vi "IQxstream_Init.vi"(4 "WaveformBW":u16(ring)=1 items=["20 MHz", "100 MHz"], 6 "Transmission":u16(ring) items=["CW", "Waveform"], 8 "error in (no error)":errorcluster, 9 "TRXmode":u16(ring) items=["Tx", "Rx"], 10 "Freq":dbl=3.5 format="%#_13g", 11 "VISA resource name":refnum<visa-resource-name>="LitePoint_IQxstream") -> (0 "error out":errorcluster, 2 "read buffer":string="LitePoint,IQxstream-5G,IQ132CA8300,1.11.2\n", 3 "VISA resource name out":refnum<visa-resource-name>="LitePoint_IQxstream")   [LabVIEW 2020, in "LitePoints.lvlib"]
uses:
  LitePoints.lvlib
panel:
  # "GHz"
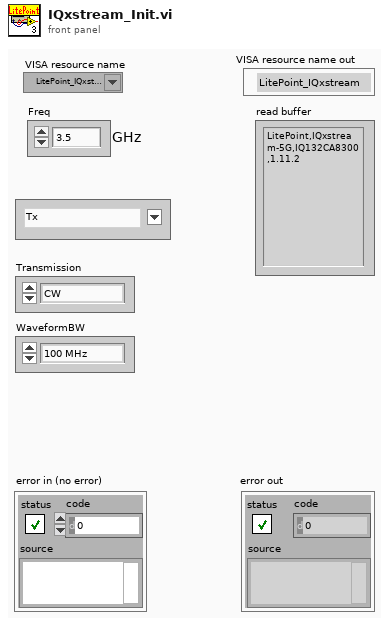
[diagram p1: front panel]
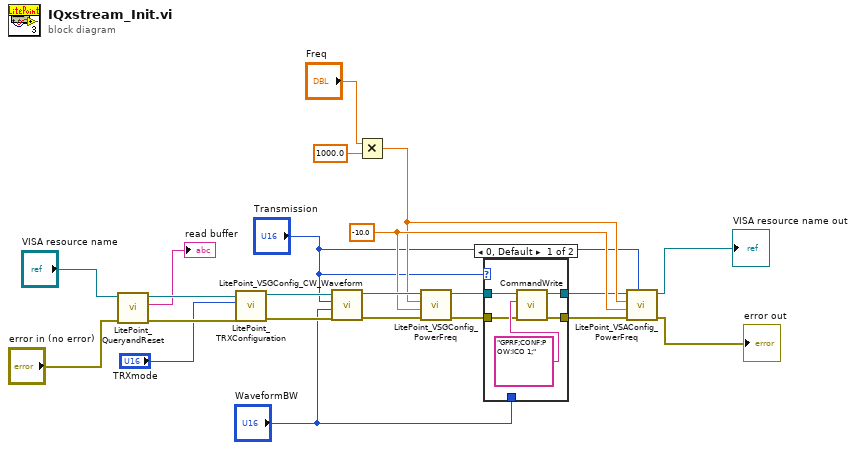
[diagram p0: block diagram]
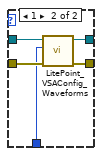
[diagram p2: hidden frame]
diagram:
  w10 = -10.0 ("Power")
  n1 = call "LitePoint_QueryandReset.vi"("error in (no error)"="error in (no error)", "VISA resource name"="VISA resource name") -> ("error out"=w20:errorcluster, "read buffer"=→"read buffer":string, "VISA resource name out"=w21:refnum<visa-resource-name>)  [unwired: 7 in]
  n2 = call "LitePoint_TRXConfiguration.vi"("error in (no error)"=w20, "TRXmode"="TRXmode", "VISA resource name"=w21) -> ("error out"=w16:errorcluster, "VISA resource name out"=w17:refnum<visa-resource-name>)  [unwired: 7 in]
  n3 = call "LitePoint_VSGConfig_CW_Waveform.vi"("error in (no error)"=w16, "WaveformBW"="WaveformBW", "Transmission"="Transmission", "VISA resource name"=w17) -> ("error out"=w15:errorcluster, "VISA resource name out"=w14:refnum<visa-resource-name>)  [unwired: 6 in]
  n4 = Multiply(x="Freq", y=1000.0) -> (x*y=w9:dbl)
  n5 = call "LitePoint_VSGConfig_PowerFreq.vi"("error in (no error)"=w15, "Power"=w10, "Freq_MHz"=w9, "VISA resource name"=w14) -> ("error out"=w5:errorcluster, "VISA resource name out"=w6:refnum<visa-resource-name>)  [unwired: 6 in]
  n6 = case shown="0, Default" "Transmission" {
    tunnel: w6 -> [w25 w32]
    tunnel: w5 -> [w26 w31]
    tunnel: [w23 w30] -> w4
    tunnel: [w24 w29] -> w3
    tunnel: "WaveformBW" -> [_ w28]
    frame 0, Default {
      n7 = call "CommandWrite.vi"("error in (no error)"=w26, "Write Buffer"="GPRF;CONF:POW:ICO 1;", "VISA resource name"=w25) -> ("error out"=w23:errorcluster, "VISA resource name out"=w24:refnum<visa-resource-name>)  [unwired: 7 in]
    }
    frame 1 {
      n8 = call "LitePoint_VSAConfig_Waveforms.vi"("error in (no error)"=w31, "WaveformBW"=w28, "VISA resource name"=w32) -> ("error out"=w30:errorcluster, "VISA resource name out"=w29:refnum<visa-resource-name>)  [unwired: 7 in]
    }
  }
  n9 = call "LitePoint_VSAConfig_PowerFreq.vi"("Transmission"="Transmission", "error in (no error)"=w4, "Power"=w10, "Freq_MHz"=w9, "VISA resource name"=w3) -> ("error out"=→"error out":errorcluster, "VISA resource name out"=→"VISA resource name out":refnum<visa-resource-name>)  [unwired: 5 in]
